vi "GraphHeight(SubVI).vi"(8 "Error In":errorcluster, 10 "XYGraph in":refnum<vi>, 11 "This VI":refnum<vi>) -> (0 "Error Out":errorcluster)   [LabVIEW 2018]
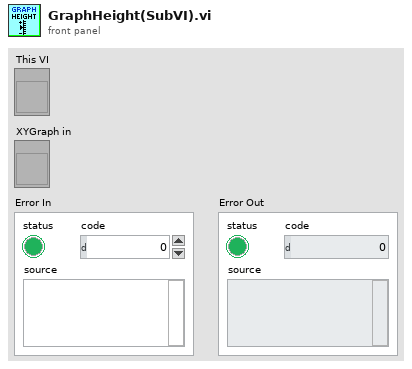
[diagram p1: front panel]
types:
  T1 = typedef "LVRectTypeDef.ctl" = cluster{"Left":i16, "Top":i16, "Right":i16, "Bottom":i16}
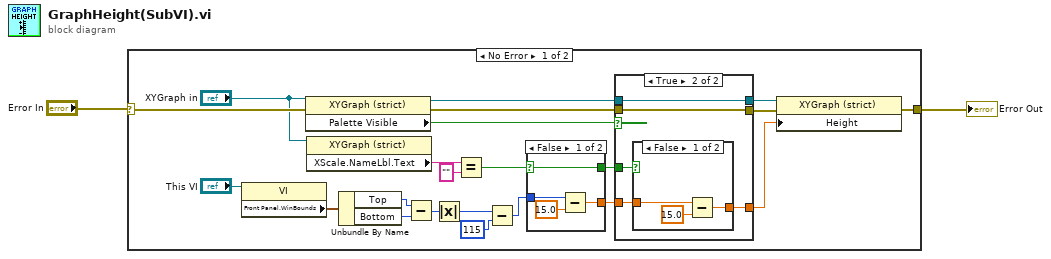
[diagram p0: block diagram]
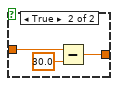
[diagram p4: hidden frame]
diagram:
  n1 = case shown="No Error" "Error In" {
    selector: "Error In" -> [w8 w45]
    tunnel: [w7 w45] -> w1
    frame No Error {
      n2 = property class="VI"(reference="This VI") -> ("Front Panel.WinBounds"=w21:T1)  [unwired: 1 in, 2 out]
      n3 = property on="Property Node" class="XYGraph (strict)"(reference="XYGraph in", error in=w8) -> (reference out=w23:refnum<vi>, error out=w22:errorcluster, "Palette Visible"=w24:bool)
      n4 = property on="Property Node" class="XYGraph (strict)"(reference="XYGraph in") -> ("XScale.NameLbl.Text"=w16:string)  [unwired: 1 in, 2 out]
      n5 = Unbundle By Name(w21) -> ("Top"=w20:i16, "Bottom"=w19:i16)
      n6 = Subtract(x=w20, y=w19) -> (x-y=w6:i16)
      n7 = Absolute Value(x=w6) -> (abs(x)=w5:i16)
      n8 = Equal?(x=w16, y="") -> (x = y?=w14:bool)
      n9 = Subtract(x=w5, y=i16 115) -> (x-y=w13:i16)
      n10 = case shown="False" w14 {
        selector: w14 -> [w25 w29]
        tunnel: w13 -> [w27 w30]
        tunnel: [w26 w30] -> w12
        tunnel: [w25 w29] -> w3
        frame False {
          n11 = Subtract(x=w27, y=15.0) -> (x-y=w26:dbl)
        }
        frame True {
        }
      }
      n12 = case shown="True" w24 {
        tunnel: w23 -> [w33 w36]
        tunnel: w22 -> [w32 w35]
        tunnel: w12 -> [w31 w38]
        tunnel: [w31 w37] -> w11
        tunnel: [w33 w36] -> w10
        tunnel: [w32 w35] -> w9
        tunnel: w3 -> [_ w34]
        frame False {
        }
        frame True {
          n13 = case shown="False" w34 {
            tunnel: w38 -> [w40 w44]
            tunnel: [w39 w42] -> w37
            frame False {
              n14 = Subtract(x=w40, y=15.0) -> (x-y=w39:dbl)
            }
            frame True {
              n15 = Subtract(x=w44, y=30.0) -> (x-y=w42:dbl)
            }
          }
        }
      }
      n16 = property on="Property Node" class="XYGraph (strict)"(reference=w10, error in=w9, "Height"=w11) -> (error out=w7:errorcluster)  [unwired: 1 out]
    }
    frame Error {
    }
  }
  "Error Out" <- w1
